vi "LVObject to JSON - Error Input - Returns Empty String.vi"() -> ()   [LabVIEW 2017, in "JSON Serializable Serializer Tests.lvlib"]
uses:
  JSON Serializable Serializer Tests.lvlib
  JSON Serializable Serializer/JSON Serializable Serializer.lvclass
  <vilib>/Utility/error.llb/Error Cluster From Error Code.vi
  <vilib>/addons/_JKI Toolkits/Caraya/classes/Assert/Assert Equal Value_Variant.vi
  <vilib>/ErrorRing/Error Ring.xnode
  <vilib>/addons/_JKI Toolkits/Caraya/classes/Test/Test.lvclass
  <vilib>/addons/_JKI Toolkits/Caraya/classes/Assert/Assert.lvclass
  Mock JSON Serializable/Mock JSON Serializable.lvclass
panel:
  out "error out":errorcluster
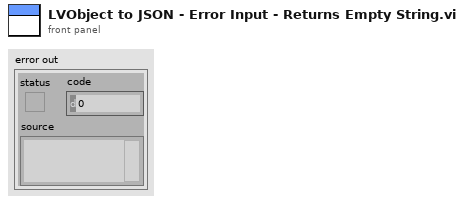
[diagram p1: front panel]
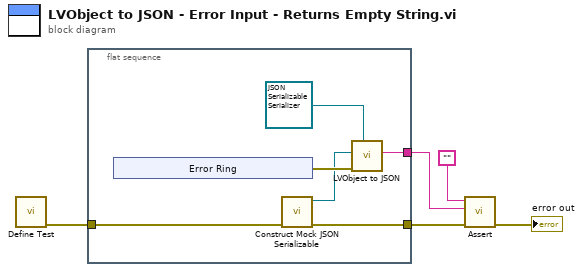
[diagram p0: block diagram]
diagram:
  n1 = call <vilib>:"Define Test.vi"() -> ("error out"=w3:errorcluster)  [unwired: 11 in]
  n2 = flat-sequence {
    tunnel: [w8] -> w5
    tunnel: [w7] -> w4
    tunnel: w3 -> [w10]
    frame #0 {
      n3 = xnode "Error Ring"() -> ("error out"=w11:errorcluster)
      n4 = call "Construct Mock JSON Serializable.vi"("error in (no error)"=w10) -> ("error out"=w7:errorcluster, "Mock JSON Serializable"=w6:refnum<class "Mock JSON Serializable.lvclass">)  [unwired: 9 in]
      n5 = call-dynamic "LVObject to JSON.vi"("JSON Serializer in"=refnum<class "JSON Serializable Serializer.lvclass"> refnum ("JSON Serializer.lvclass"), "error in (no error)"=w11, "Object"=w6) -> ("<JSON>Object"=w8:string)  [unwired: 7 in, 1 out]
    }
  }
  n6 = call-poly <vilib>:"Assert.vi"("error in (no error)"=w4, "Y"=w5, "X"="") -> ("error out"=→"error out":errorcluster)  [unwired: 8 in]
